vi "Arm Motors.vi"() -> ()   [LabVIEW 2018]
uses:
  <vilib>/Rock Robotics/WPI/ThirdParty/Phoenix-LabVIEW/Motor Controller/Controls/CTRE_Phoenix_MotorControl_NeutralMode.ctl
  <vilib>/Rock Robotics/WPI/ThirdParty/Phoenix-LabVIEW/Motor Controller/Controls/CTRE_Phoenix_MotorControl_ControlMode.ctl
  Framework/Robot Global Data.vi
  <vilib>/ptbypt/NI_PtbyPt.lvlib
panel:
  out "Override Limit":bool
  in  "Override Limit":bool
  out "Current Angle":dbl
  out "Loop Count":i32
  in  "Drop-Off Angle":dbl=110.0
  out "Waveform Chart":T1(graph)
  in  "Proportional Slowdown":dbl=40.0
  in  "Min speed":dbl=0.06 min=0.0 max=1.0 step=0.01
  out "Arm Angle Error":dbl format="%.2f"
  in  "Motor Tuning":T2={"Max Motor Speed"=1.0, "Decel Angle (Deg)"=40.0, "Deadband Angle (Deg)"=0.5} {"Max Motor Speed" min=0.0 max=1.0 step=0.05}
  in  "Loop Time":u32=20
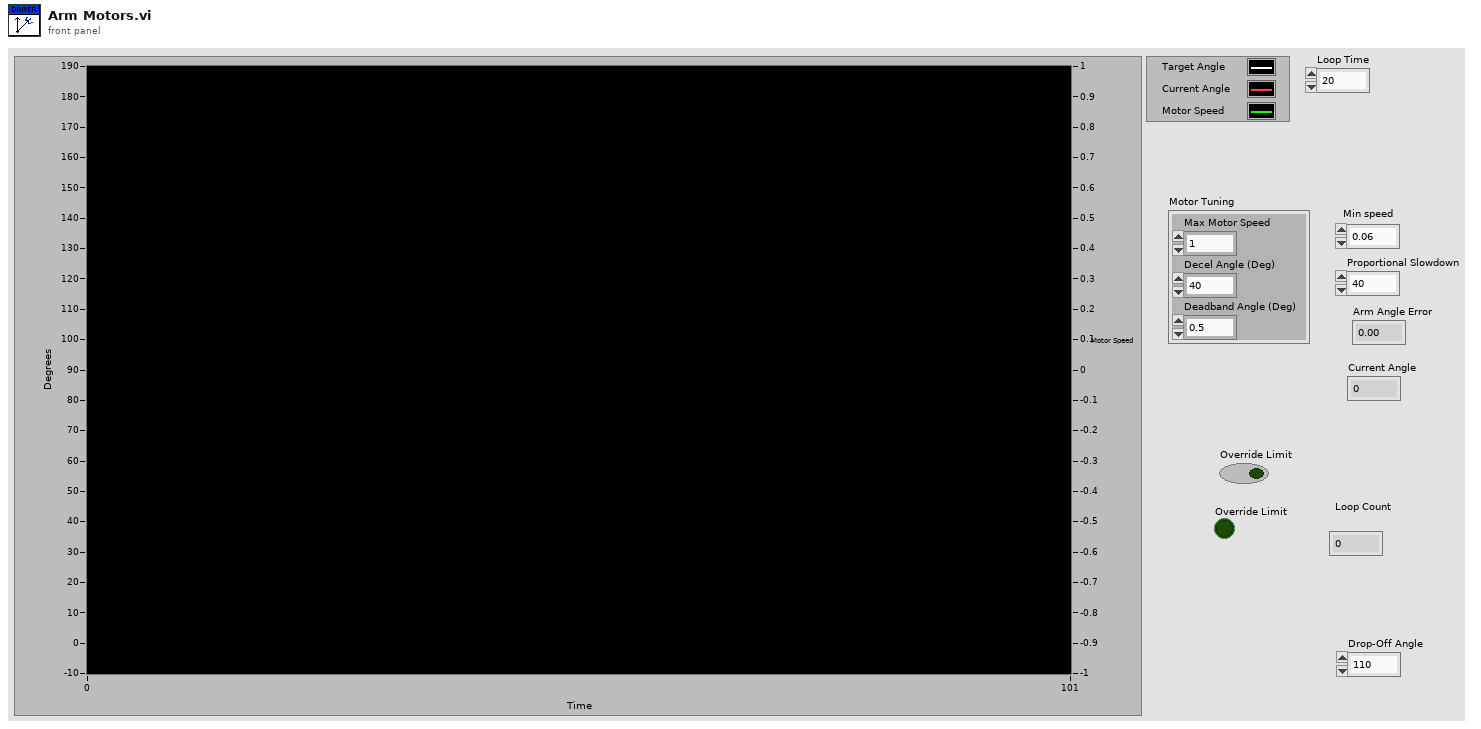
[diagram p1: front panel]
types:
  T1 = cluster{"Target Angle":dbl, "Current Angle":dbl, "Motor Speed":dbl}[]
  T2 = cluster{"Max Motor Speed":dbl, "Decel Angle (Deg)":dbl, "Deadband Angle (Deg)":dbl}
  T3 = typedef "CTRE_Phoenix_MotorControl_NeutralMode.ctl" = enum8{"EEPROMSetting", "Override to Coast", "Override to Brake"}
  T4 = typedef "WPI_MotorControlDeviceRef.ctl" = cluster{"DeviceStatus":errorcluster, "Type":T5, "PWM":cluster{"PWM Channel":T6, "DeadBand":T7}, "CAN":cluster{"Device Number":u8, "SetOutput VI Ref":variant, "GetOutput VI Ref":variant, "Enable VI Ref":variant, "Disable VI Ref":variant, "Data":variant}, "Invert":bool, "DIO PWM":cluster{"PWM \"Enable\" Channel":T6, "DIOChannel":T8, "PWM Rate":dbl}}
  T5 = typedef "WPI_MotorControlType.ctl" = enum16{"PWM", "CAN", "DIO PWM"}
  T6 = typedef "FPGA_DIOPWMChannel.ctl" = enum8{"PWM 0", "PWM 1", "PWM 2", "PWM 3", "PWM 4", "PWM 5", "PWM 6", "PWM 7", "PWM 8", "PWM 9", "PWM MXP 0", "PWM MXP 1", "PWM MXP 2", "PWM MXP 3", "PWM MXP 4", "PWM MXP 5", "PWM MXP 6", "PWM MXP 7", "PWM MXP 8", "PWM MXP 9", "Invalid"}
  T7 = typedef "WPI_PWMDeadband.ctl" = cluster{"Name":string, "maxPositivePwm":i32, "minPositivePwm":i32, "centerPwm":i32, "maxNegativePwm":i32, "minNegativePwm":i32, "angularRange":u16}
  T8 = typedef "FPGA_DIOChannel.ctl" = enum8{"DIO 0", "DIO 1", "DIO 2", "DIO 3", "DIO 4", "DIO 5", "DIO 6", "DIO 7", "DIO 8", "DIO 9", "DIO MXP 0", "DIO MXP 1", "DIO MXP 2", "DIO MXP 3", "DIO MXP 4", "DIO MXP 5", "DIO MXP 6", "DIO MXP 7", "DIO MXP 8", "DIO MXP 9", "DIO MXP 10", "DIO MXP 11", "DIO MXP 12", "DIO MXP 13", "DIO MXP 14", "DIO MXP 15", "SPI Port CS1", "SPI Port CS2", "SPI Port CS3", "SPI Port MISO", "SPI Port MOSI", "Invalid"}
  T9 = cluster{"Target Angle":dbl, "Current Angle":dbl, "Motor Speed":dbl}
  T10 = typedef "WPI_DriverStationRobotMode2.ctl" = enum16{"Autonomous Disabled", "Autonomous Enabled", "Teleop Disabled", "Teleop Enabled", "Disconnected", "Finish", "Test Disabled", "Test Enabled", "Emergency Stopped"}
  T11 = typedef "CTRE_Phoenix_MotorControl_ControlMode.ctl" = u16
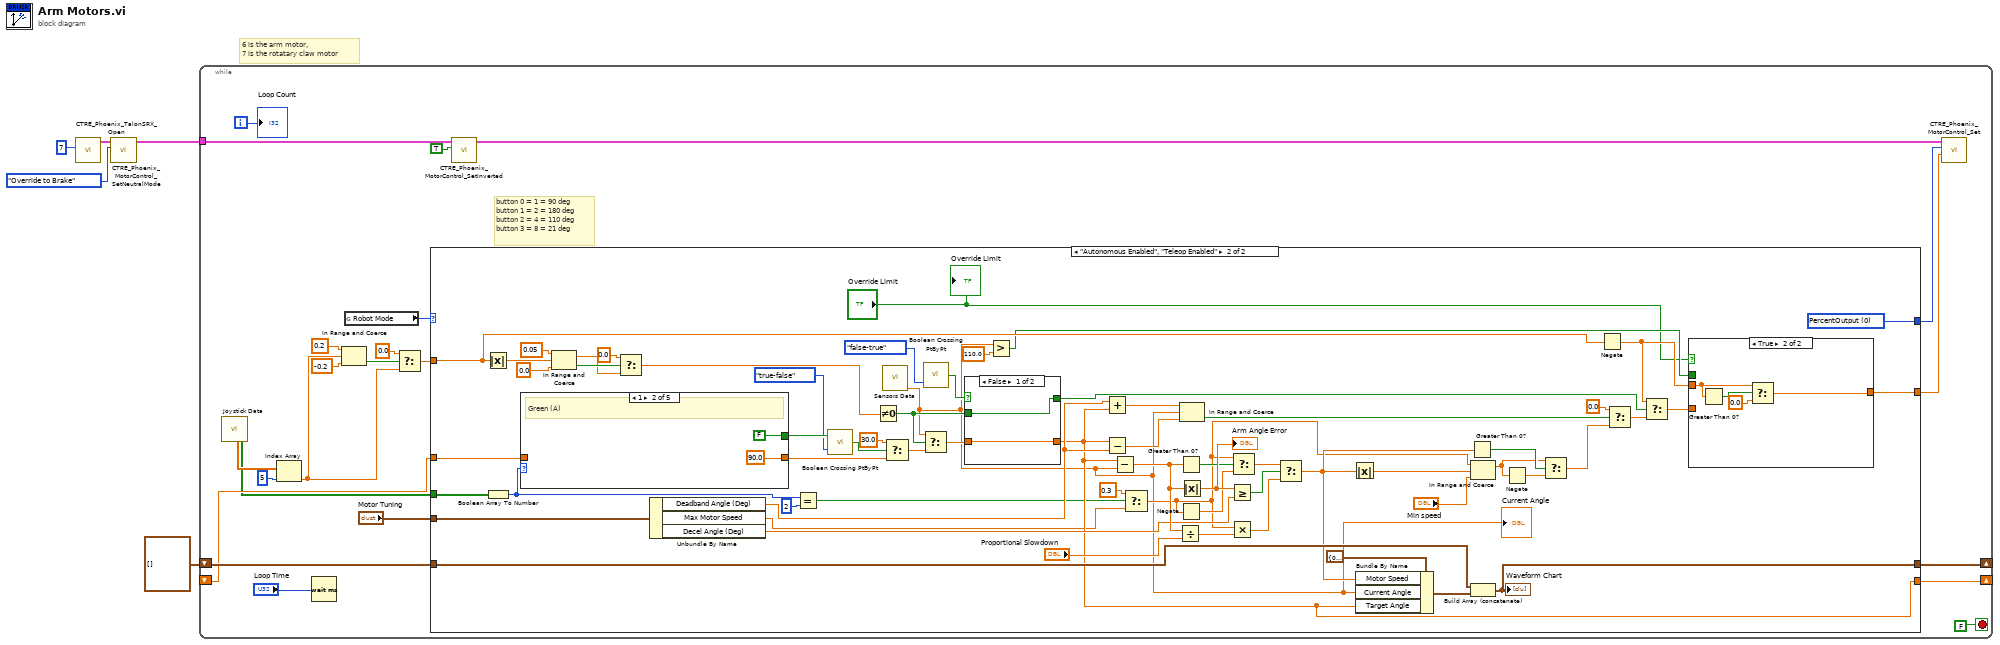
[diagram p0: block diagram]
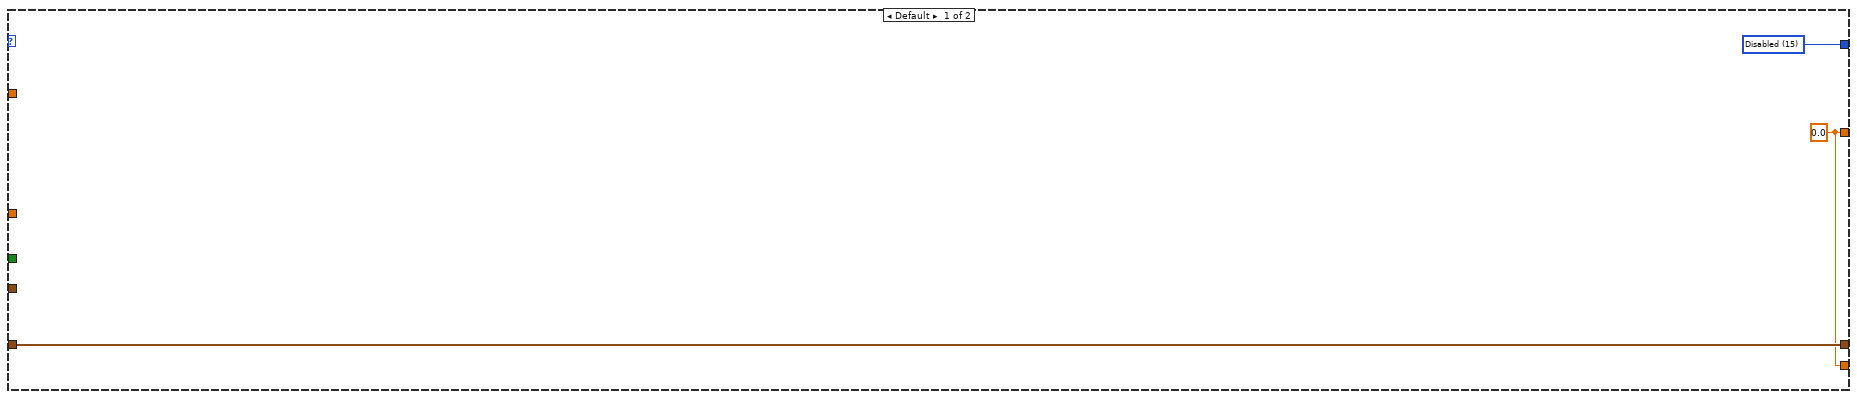
[diagram p2: hidden frame]
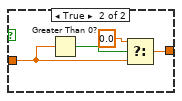
[diagram p4: hidden frame]
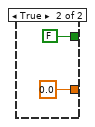
[diagram p5: hidden frame]
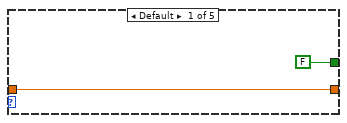
[diagram p6: hidden frame]
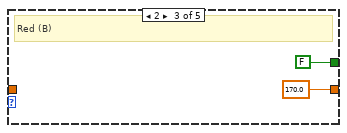
[diagram p7: hidden frame]
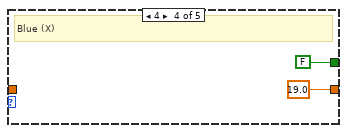
[diagram p8: hidden frame]
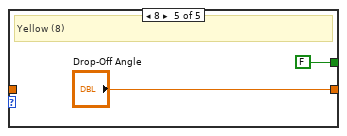
[diagram p9: hidden frame]
diagram:
  # "6 is the arm motor, \n7 is the rotatary claw motor"
  n1 = call <vilib>:"CTRE_Phoenix_TalonSRX_Open.vi"("Device Number"=7) -> ("CAN Talon SRX Ref"=w4:T4)  [unwired: 9 in, 1 out]
  n2 = call <vilib>:"CTRE_Phoenix_MotorControl_SetNeutralMode.vi"("Motor Control Neutral Mode"=CTRE_Phoenix_MotorControl_NeutralMode."Override to Brake", "PhoenixMotorControlDevRef"=w4) -> ("PhoenixMotorControlDevRef"=w1:T4)  [unwired: 8 in, 1 out]
  n3 = while {
    tunnel: w1 -> [w21]
    shift-right: [w24] -> _
    shift-left: T1 [] -> [w25]
    shift-right: [w20] -> _
    shift-left: _ -> [w19]
    i -> [w6]
    stop <- FALSE stop-if-true
    # "button 0 = 1 = 90 deg\nbutton 1 = 2 = 180 deg\nbutton 2 = 4 = 110 deg\nbutton 3 = 8 = 21 deg"
    n4 = call "Joystick Data.vi"() -> ("Xbox 360 Joy Out"=w8:dbl[], "Xbox 360 Out"=w7:bool[])  [unwired: 12 in, 6 out]
    n5 = Index Array(array=w8, index=5) -> (element=w9:dbl)
    n6 = Wait (ms)(milliseconds to wait="Loop Time") -> ()  [unwired: 1 out]
    n7 = In Range and Coerce(upper limit=0.2, x=w9, lower limit=-0.2) -> (In Range?=w12:bool)  [unwired: 1 out]
    n8 = global read "Robot Global Data.vi" "Robot Mode"() -> (w28:T10)
    n9 = Select(t=0.0, s=w12, f=w9) -> (s? t:f=w13:dbl)
    n10 = case shown="\"Autonomous Enabled\", \"Teleop Enabled\"" w28 {
      tunnel: [w31 w82] -> w18
      tunnel: [w29 w44] -> w16
      tunnel: w25 -> [w30 w86]
      tunnel: [w30 w84] -> w24
      tunnel: "Motor Tuning" -> [_ w62]
      tunnel: w7 -> [_ w71]
      tunnel: [w29 w63] -> w20
      tunnel: w19 -> [_ w69]
      tunnel: w13 -> [_ w52]
      frame Default {
        w31 = T11 15 items=["PercentOutput"=0, "Position"=1, "Velocity"=2, "Current"=3, "Follower"=5, "MotionProfile"=6, "MotionMagic"=7, "MotionProfileArc"=10, "Disabled"=15] ("Control Mode")
        w29 = 0.0 ("f")
      }
      frame "Autonomous Enabled", "Teleop Enabled" {
        w82 = T11 0 items=["PercentOutput"=0, "Position"=1, "Velocity"=2, "Current"=3, "Follower"=5, "MotionProfile"=6, "MotionMagic"=7, "MotionProfileArc"=10, "Disabled"=15] ("Control Mode")
        n11 = Absolute Value(x=w52) -> (abs(x)=w51:dbl)
        n12 = Boolean Array To Number(Boolean array=w71) -> (number=w56:u32)
        n13 = case shown="1" w56 {
          tunnel: [w113 90.0 ("index") 170.0 ("index") 19.0 ("index") "Drop-Off Angle"] -> w39
          tunnel: w69 -> [w113 _ _ _ _]
          tunnel: [FALSE FALSE FALSE FALSE FALSE] -> w42
          frame Default {
          }
          frame 1 {
            # "Green (A)"
          }
          frame 2 {
            # "Red (B)"
          }
          frame 4 {
            # "Blue (X)"
          }
          frame 8 {
            # "Yellow (8)"
          }
        }
        n14 = In Range and Coerce(upper limit=0.05, x=w51, lower limit=0.0) -> (coerced(x)=w47:dbl, In Range?=w48:bool)
        n15 = Select(t=0.0, s=w48, f=w47) -> (s? t:f=w45:dbl)
        n16 = Unbundle By Name(w62) -> ("Deadband Angle (Deg)"=w70:dbl, "Max Motor Speed"=w57:dbl, "Decel Angle (Deg)"=w83:dbl)
        n17 = Equal?(x=w56, y=u32 2) -> (x = y?=w60:bool)
        n18 = call <vilib>:"Boolean Crossing PtByPt.vi"("direction"=enum16{"either", "false-true", "true-false"}."true-false", "input"=w42) -> ("crossing"=w40:bool)  [unwired: 1 in]
        n19 = Not Equal To 0?(x=w45) -> (x != 0?=w53:bool)
        n20 = call "Sensors Data.vi"() -> ("Distance Out"=w33:dbl)  [unwired: 8 in, 3 out]
        "Current Angle" <- w33
        n21 = Select(t=30.0, s=w40, f=w39) -> (s? t:f=w37:dbl)
        n22 = Select(t=w33, s=w53, f=w37) -> (s? t:f=w65:dbl)
        n23 = call <vilib>:"Boolean Crossing PtByPt.vi"("direction"=enum16{"either", "false-true", "true-false"}."false-true") -> ("crossing"=w66:bool)  [unwired: 2 in]
        n24 = case shown="False" w66 {
          tunnel: w65 -> [w109 _]
          tunnel: [w109 0.0 ("t")] -> w63
          tunnel: [w108 FALSE ("Manual Target")] -> w55
          tunnel: w53 -> [w108 _]
          frame False {
          }
          frame True {
          }
        }
        n25 = Greater?(x=w33, y=110.0) -> (0:w34:bool)
        n26 = Add(x=w70, y=w63) -> (x+y=w95:dbl)
        n27 = Subtract(x=w63, y=w70) -> (x-y=w94:dbl)
        n28 = Subtract(x=w63, y=w33) -> (x-y=w88:dbl)
        n29 = Select(t=0.3, s=w60, f=w57) -> (s? t:f=w59:dbl)
        n30 = Divide(x=w88, y="Proportional Slowdown") -> (x/y=w68:dbl)
        n31 = Greater Than 0?(x=w88) -> (x > 0?=w90:bool)
        n32 = Negate(x=w59) -> (-x=w89:dbl)
        n33 = In Range and Coerce(upper limit=w95, x=w33, lower limit=w94) -> (In Range?=w72:bool)  [unwired: 1 out]
        n34 = Absolute Value(x=w88) -> (abs(x)=w93:dbl)
        "Arm Angle Error" <- w93
        n35 = Greater Or Equal?(x=w93, y=w83) -> (x >= y?=w92:bool)
        n36 = Multiply(x=w59, y=w68) -> (x*y=w78:dbl)
        n37 = Select(t=w59, s=w90, f=w89) -> (s? t:f=w91:dbl)
        n38 = Select(t=w91, s=w92, f=w78) -> (s? t:f=w64:dbl)
        n39 = Absolute Value(x=w64) -> (abs(x)=w77:dbl)
        n40 = Bundle By Name(cluster=T9 {"Target Angle"=0.0, "Current Angle"=0.0, "Motor Speed"=0.0}, "Motor Speed"=w64, "Current Angle"=w33, "Target Angle"=w63) -> (w85:T9)
        n41 = Greater Than 0?(x=w64) -> (x > 0?=w76:bool)
        n42 = In Range and Coerce(upper limit=w59, x=w77, lower limit="Min speed") -> (coerced(x)=w75:dbl)  [unwired: 1 out]
        n43 = Build Array (concatenate)(w86, w85) -> (w84:T1)
        "Waveform Chart" <- w84
        n44 = Negate(x=w75) -> (-x=w74:dbl)
        n45 = Select(t=w75, s=w76, f=w74) -> (s? t:f=w73:dbl)
        n46 = Negate(x=w52) -> (-x=w43:dbl)
        n47 = Select(t=0.0, s=w72, f=w73) -> (s? t:f=w54:dbl)
        n48 = Select(t=w43, s=w55, f=w54) -> (s? t:f=w36:dbl)
        n49 = case shown="True" "Override Limit" {
          tunnel: w43 -> [_ w104]
          tunnel: [w97 w106] -> w44
          tunnel: w36 -> [w98 _]
          tunnel: w34 -> [w96 _]
          frame False {
            n50 = case shown="False" w96 {
              tunnel: w98 -> [w99 w101]
              tunnel: [w99 w100] -> w97
              frame False {
              }
              frame True {
                n51 = Greater Than 0?(x=w101) -> (x > 0?=w103:bool)
                n52 = Select(t=0.0, s=w103, f=w101) -> (s? t:f=w100:dbl)
              }
            }
          }
          frame True {
            n53 = Greater Than 0?(x=w104) -> (x > 0?=w105:bool)
            n54 = Select(t=w104, s=w105, f=0.0) -> (s? t:f=w106:dbl)
          }
        }
        "Override Limit" <- "Override Limit"
      }
    }
    n55 = call <vilib>:"CTRE_Phoenix_MotorControl_SetInverted.vi"("Invert?"=TRUE, "PhoenixMotorControlDevRef"=w21) -> ("PhoenixMotorControlDevRef"=w17:T4)  [unwired: 8 in, 1 out]
    n56 = call <vilib>:"CTRE_Phoenix_MotorControl_Set.vi"("Output"=w16, "Control Mode"=w18, "PhoenixMotorControlDevRef"=w17) -> ()  [unwired: 7 in, 2 out]
    "Loop Count" <- w6
  }
